vi "Leggi perdite di carico.vi"(4 "Lungh tubo asp":dbl, 5 "Dia ASP":string, 6 "Enum":T1(ring), 7 "Dia mand":string, 8 "PORTATA":dbl, 9 "DIAMETRO MAND ASP":i16, 10 "TAGLIA":string, 11 "SERIE":string) -> (0 "Perdite carico Mandata":dbl, 1 "Perdite carico Misura":dbl, 2 "Perdite carico MAND":dbl, 3 "Perdite carico ASP":dbl)   [LabVIEW 2019]
uses:
  Global percorso impostazioni.vi
panel:
  in  "Excel._Worksheet 15":refnum<k7>
  in  "Excel._Worksheet 14":refnum<k7>
  in  "Excel._Worksheet 13":refnum<k7>
  in  "Excel._Worksheet 12":refnum<k7>
  in  "Excel._Worksheet 10":refnum<k7>
  in  "Excel._Worksheet 4":refnum<k7>
  in  "WindowState 3":i32(ring)=-4137 items=["xlMaximized"=-4137, "xlMinimized"=-4140, "xlNormal"=-4143]
  out "error out 2":errorcluster
  in  "Excel._Worksheet 9":refnum<k7>
  in  "Excel._Worksheet 8":refnum<k7>
  out "error out":errorcluster
  in  "Excel._Worksheet 7":refnum<k7>
  in  "Excel._Worksheet 6":refnum<k7>
  in  "Excel._Worksheet 5":refnum<k7>
  in  "Excel._Worksheet 3":refnum<k7>
  in  "Excel._Worksheet 2":refnum<k7>
  in  "WindowState 2":i32(ring)=-4137 items=["xlMaximized"=-4137, "xlMinimized"=-4140, "xlNormal"=-4143]
  # "pompe di superficie"
  # "pompe di verticali\\sommerse"
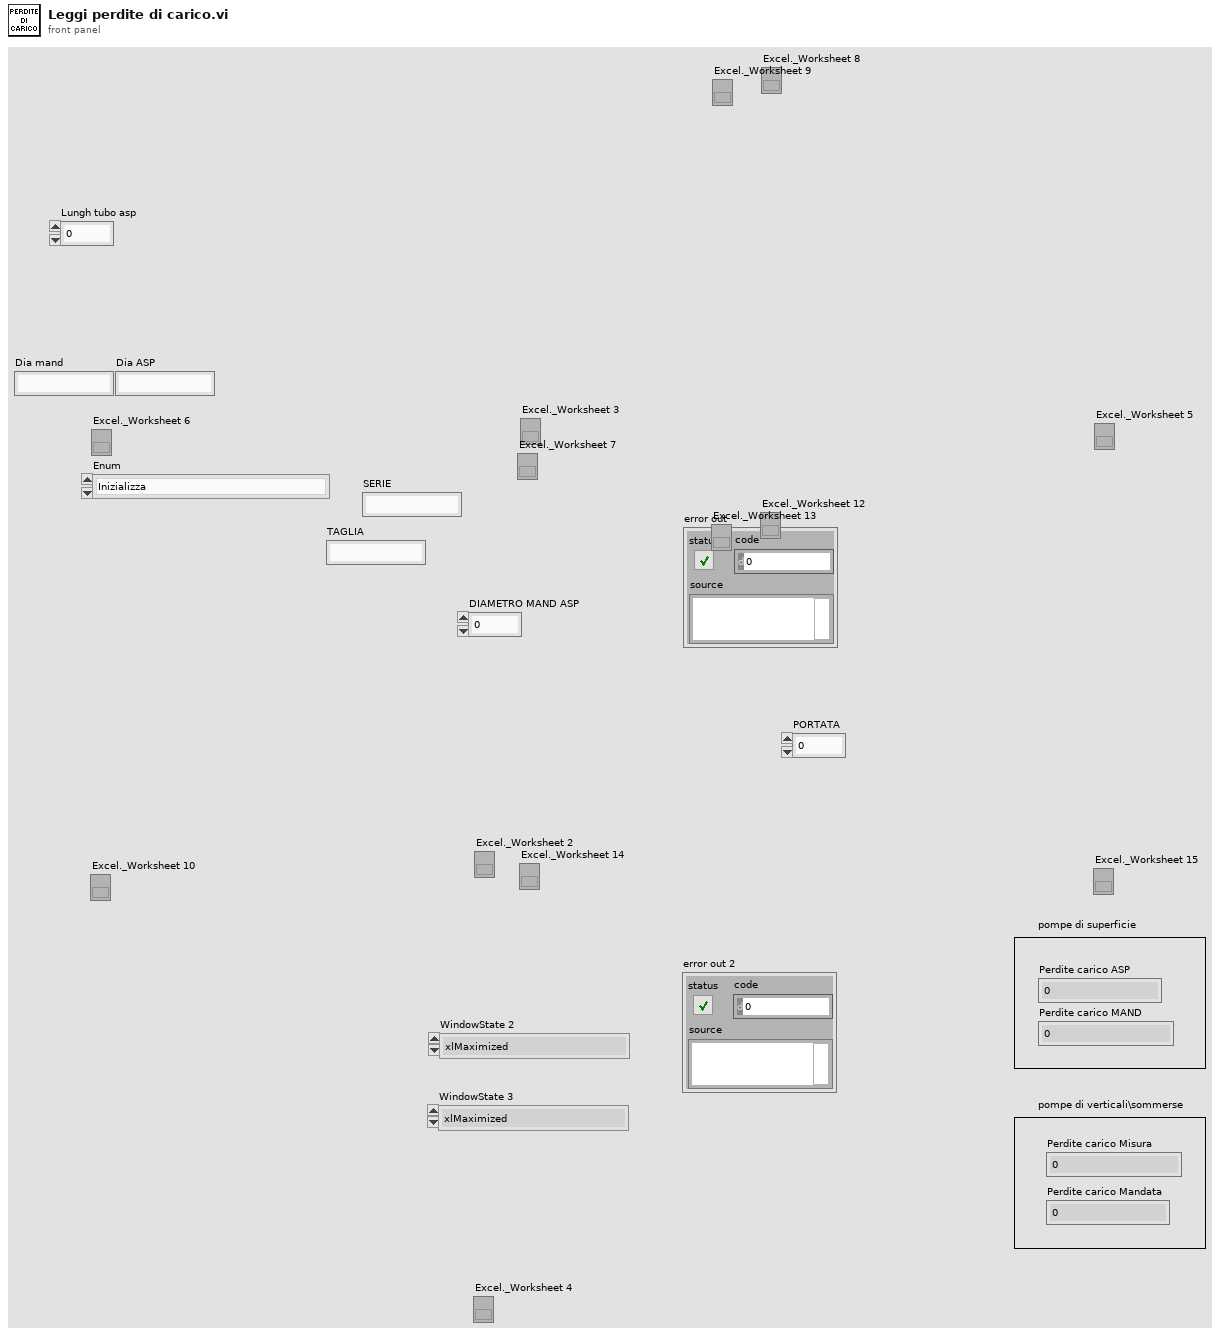
[diagram p1: front panel]
types:
  T1 = enum16{"Inizializza", "Imposta selezioni pompa", "Leggi perdite", "Close"}
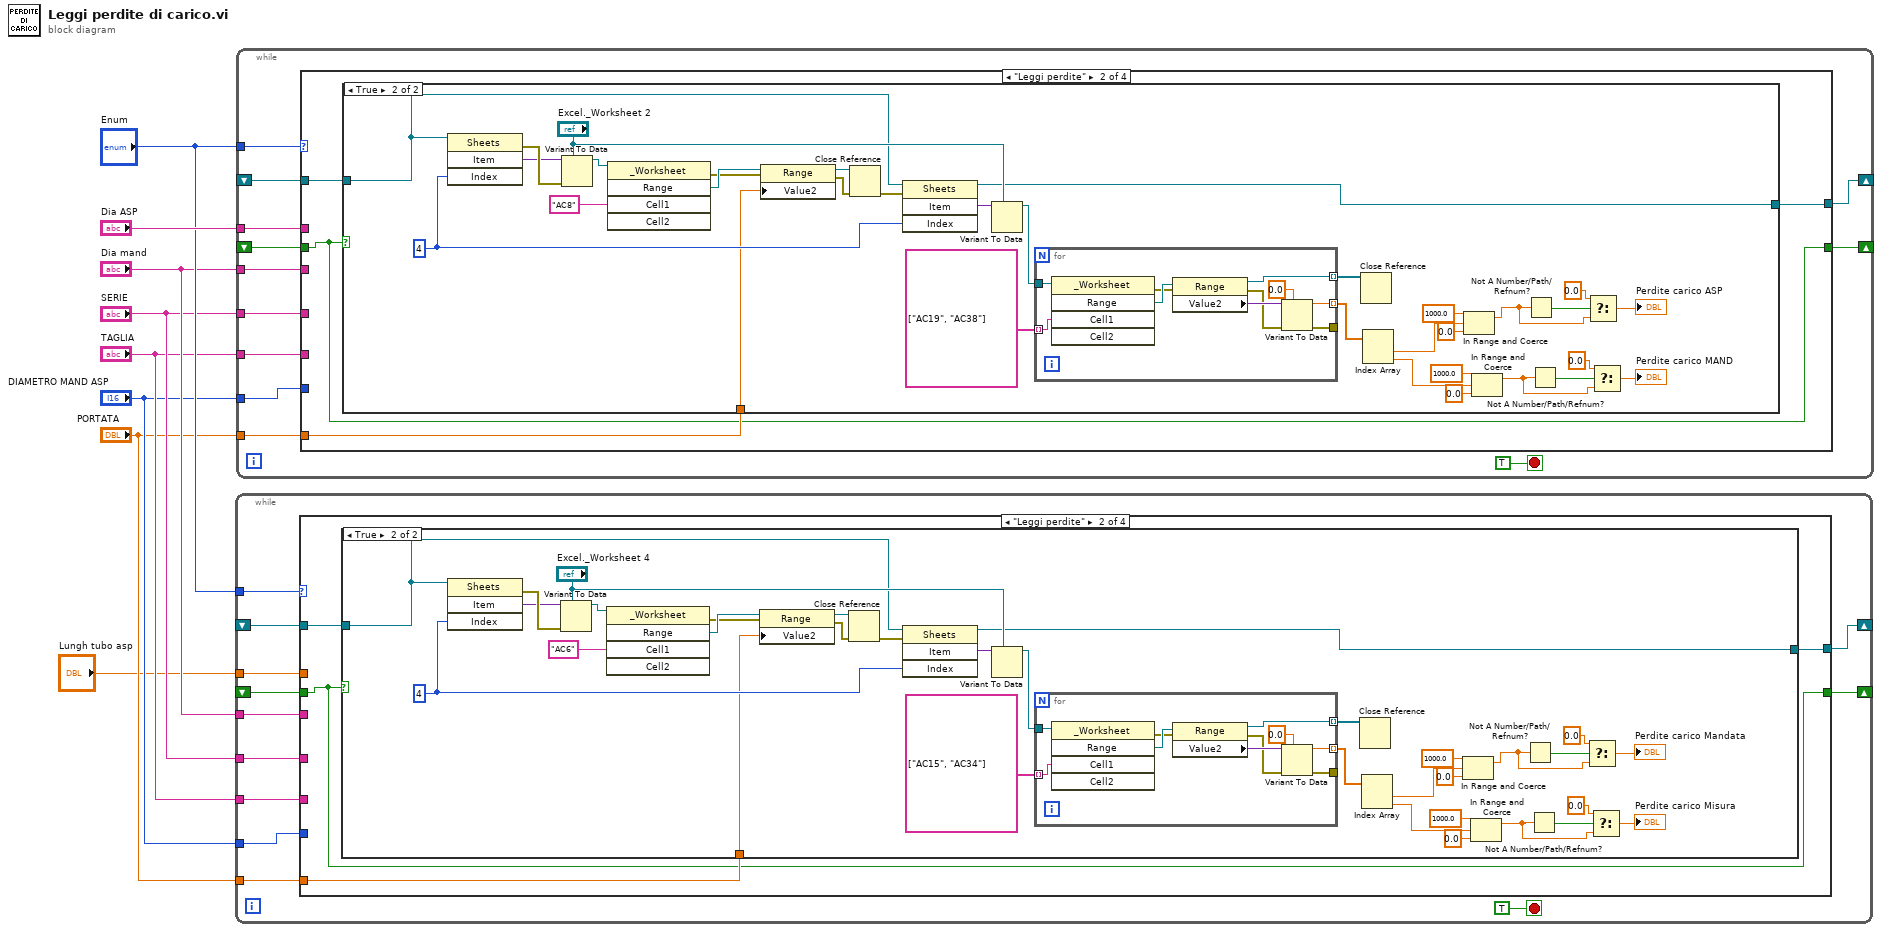
[diagram p0: block diagram]
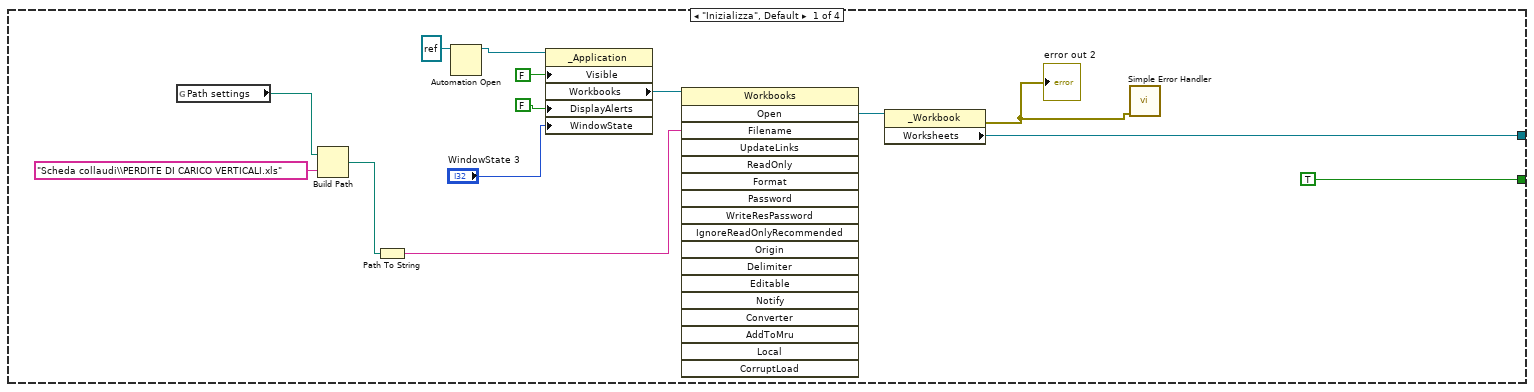
[diagram p2: hidden frame]
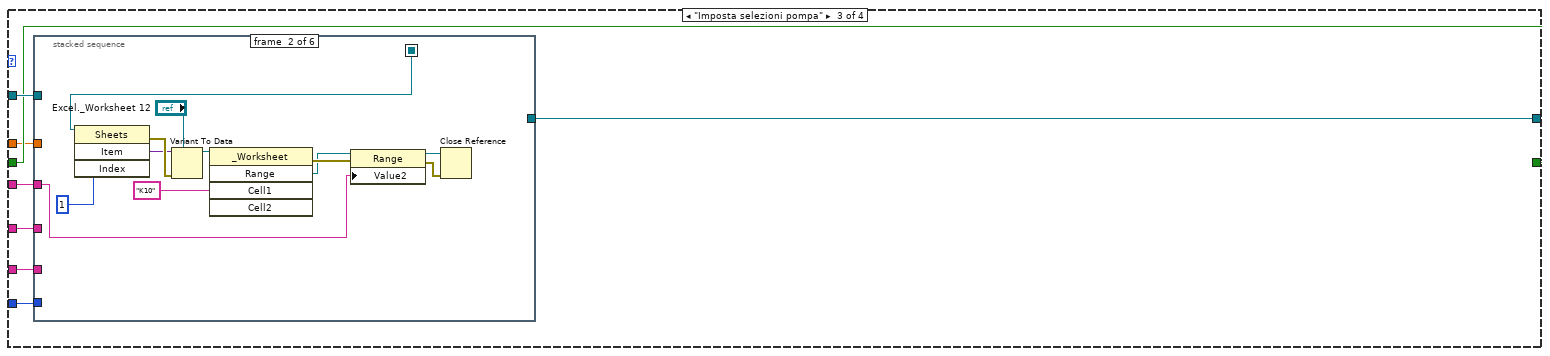
[diagram p4: hidden frame]
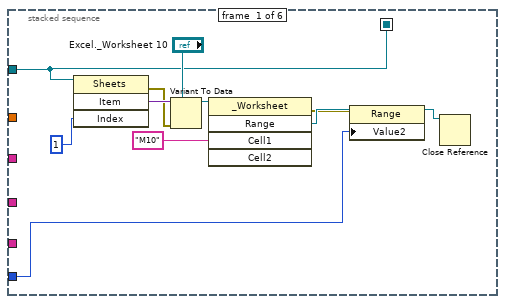
[diagram p5: hidden frame]
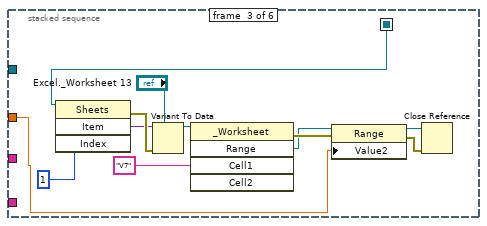
[diagram p6: hidden frame]
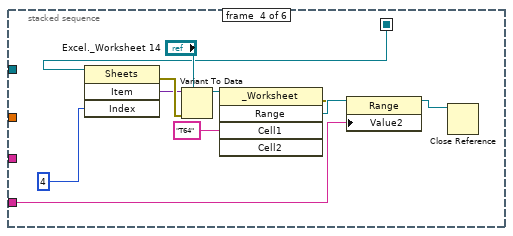
[diagram p7: hidden frame]
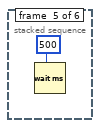
[diagram p8: hidden frame]
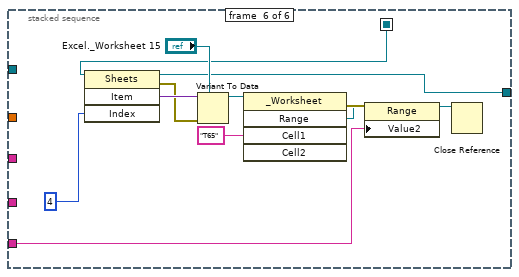
[diagram p9: hidden frame]
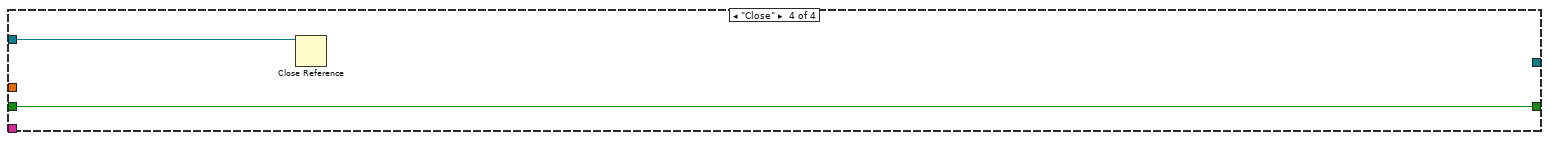
[diagram p10: hidden frame]
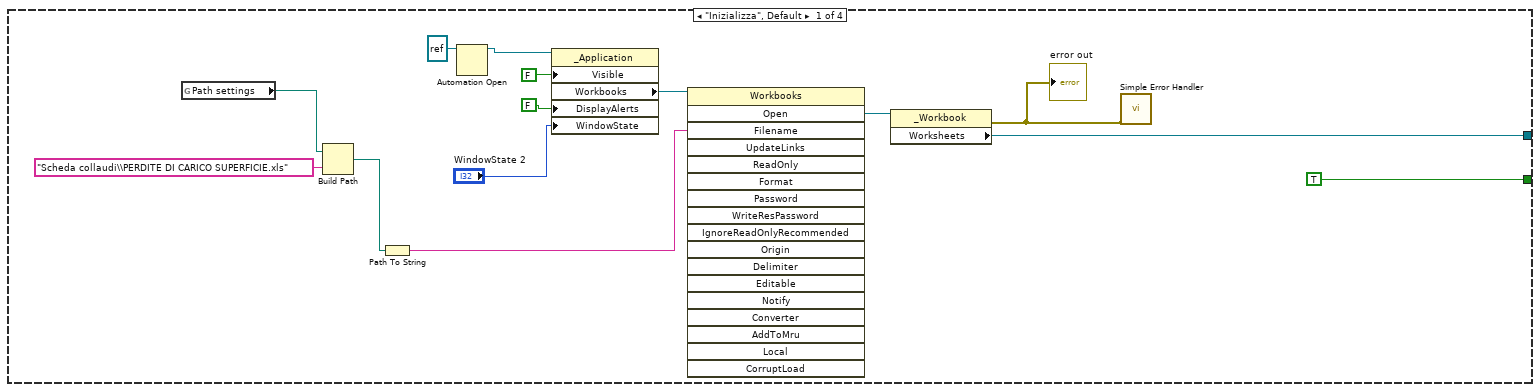
[diagram p11: hidden frame]
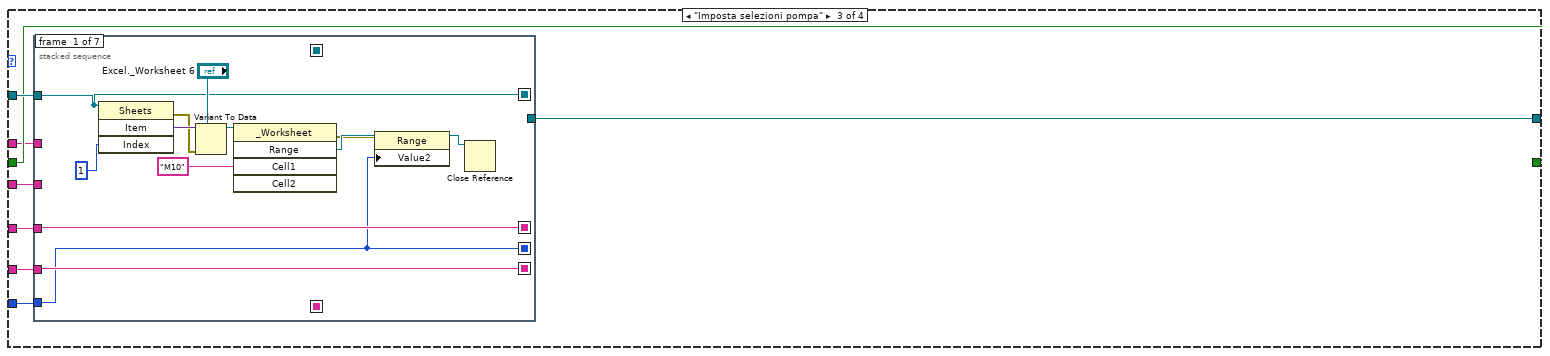
[diagram p13: hidden frame]
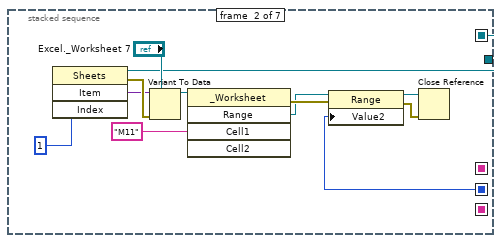
[diagram p14: hidden frame]
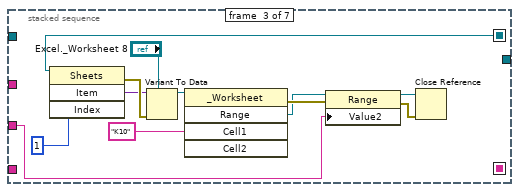
[diagram p15: hidden frame]
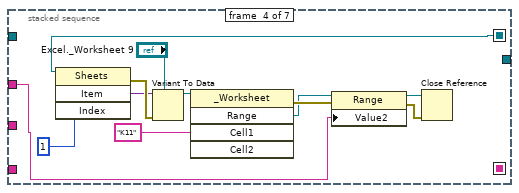
[diagram p16: hidden frame]
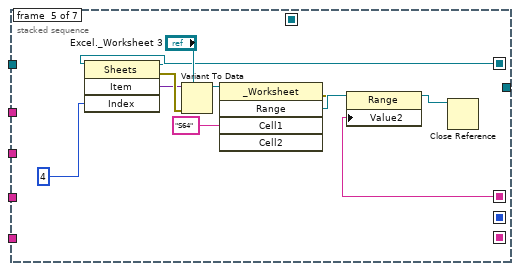
[diagram p17: hidden frame]
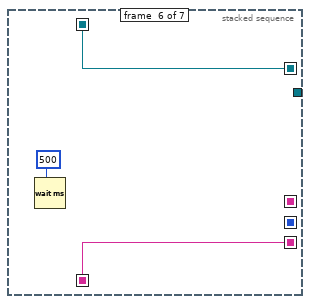
[diagram p18: hidden frame]
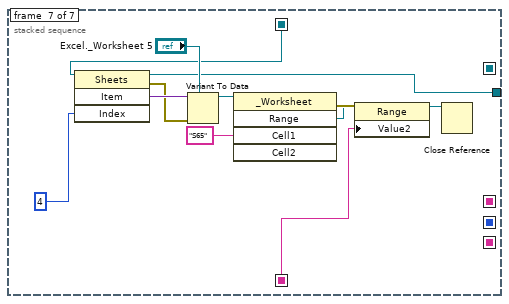
[diagram p19: hidden frame]
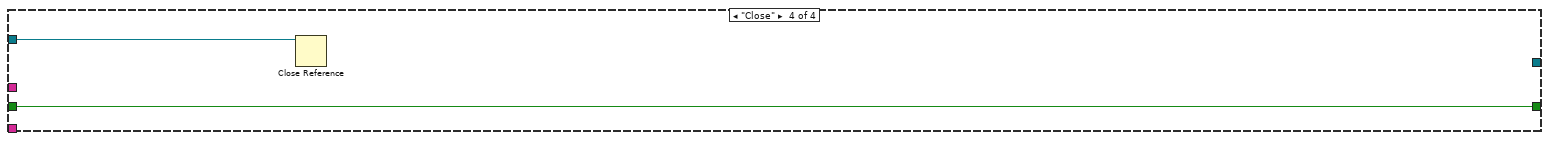
[diagram p20: hidden frame]
diagram:
  n1 = while {
    shift-right: [w19] -> _
    shift-left: _ -> [w18]
    tunnel: "SERIE" -> [w17]
    tunnel: "TAGLIA" -> [w16]
    tunnel: "DIAMETRO MAND ASP" -> [w15]
    tunnel: "Enum" -> [w14]
    tunnel: "PORTATA" -> [w13]
    shift-right: [w12] -> _
    shift-left: _ -> [w11]
    tunnel: "Dia mand" -> [w10]
    tunnel: "Lungh tubo asp" -> [w9]
    stop <- TRUE stop-if-true
    n2 = case shown="\"Leggi perdite\"" w14 {
      tunnel: [w23 w37 w86 _] -> w19
      tunnel: w18 -> [_ w38 w90 w151]
      tunnel: w17 -> [_ _ w89 _]
      tunnel: w16 -> [_ _ w88 _]
      tunnel: w15 -> [_ _ w87 _]
      tunnel: w13 -> [_ w36 _ _]
      tunnel: [TRUE w35 w85 w150] -> w12
      tunnel: w11 -> [_ w35 w85 w150]
      tunnel: w10 -> [_ _ w84 _]
      tunnel: w9 -> [_ _ w83 _]
      frame "Inizializza", Default {
        n3 = global read "Global percorso impostazioni.vi" "Path settings"() -> (w27:path)
        n4 = Build Path(base path=w27, name or relative path="Scheda collaudi\\PERDITE DI CARICO VERTICALI.xls") -> (appended path=w25:path)
        n5 = Path To String(path=w25) -> (string=w33:string)
        n6 = Automation Open(Automation Refnum=refnum<k7> refnum ("Excel._Application")) -> (Automation Refnum=w34:refnum<k7>)  [unwired: 3 in, 1 out]
        n7 = property class="_Application"(reference=w34, "Visible"=FALSE, "DisplayAlerts"=FALSE, "WindowState"="WindowState 3") -> ("Workbooks"=w22:refnum<k7>)  [unwired: 1 in, 2 out]
        n8 = invoke class="Workbooks" method="Open"(reference=w22, "Filename"=w33) -> ("Open"=w24:refnum<k7>)  [unwired: 16 in, 17 out]
        n9 = property class="_Workbook"(reference=w24) -> (error out=w21:errorcluster, "Worksheets"=w23:refnum<k7>)  [unwired: 1 in, 1 out]
        "error out 2" <- w21
        n10 = call <vilib>:"Simple Error Handler.vi"("error in (no error)"=w21) -> ()  [unwired: 4 in, 5 out]
      }
      frame "Leggi perdite" {
        n11 = case shown="True" w35 {
          tunnel: w38 -> [w39 w58]
          tunnel: [w39 w57] -> w37
          tunnel: w36 -> [_ w40]
          frame False {
          }
          frame True {
            w64 = 4 ("Sheet Index")
            n12 = invoke class="Sheets" method="Item"(reference=w58, "Index"=w64) -> (error out=w60:errorcluster, "Item"=w59:variant)  [unwired: 2 in, 2 out]
            n13 = Variant To Data(error in=w60, type="Excel._Worksheet 4", Variant=w59) -> (data=w62:refnum<k7>)  [unwired: 1 out]
            n14 = invoke class="_Worksheet" method="Range"(reference=w62, "Cell1"="AC6") -> (error out=w65:errorcluster, "Range"=w66:refnum<k7>)  [unwired: 3 in, 3 out]
            n15 = property class="Range"(reference=w66, error in=w65, "Value2"=w40) -> (reference out=w70:refnum<k7>, error out=w71:errorcluster)
            n16 = Close Reference(reference=w70, error in (no error)=w71) -> (error out=w72:errorcluster)
            n17 = invoke class="Sheets" method="Item"(reference=w58, error in=w72, "Index"=w64) -> (reference out=w57:refnum<k7>, "Item"=w63:variant)  [unwired: 1 in, 2 out]
            n18 = Variant To Data(type="Excel._Worksheet 4", Variant=w63) -> (data=w69:refnum<k7>)  [unwired: 1 in, 1 out]
            n19 = for {
              tunnel: w69 -> [w82]
              tunnel: [w77] -> w55 mode=indexing
              tunnel: string[] ["AC15", "AC34"] -> [w76] mode=indexing
              tunnel: [w74] -> _
              tunnel: [w73] -> w56 mode=indexing
              n20 = invoke class="_Worksheet" method="Range"(reference=w82, "Cell1"=w76) -> (error out=w80:errorcluster, "Range"=w81:refnum<k7>)  [unwired: 3 in, 3 out]
              n21 = property class="Range"(reference=w81, error in=w80) -> (reference out=w73:refnum<k7>, error out=w78:errorcluster, "Value2"=w79:variant)
              n22 = Variant To Data(error in=w78, type=0.0, Variant=w79) -> (data=w77:dbl, error out=w74:errorcluster)
            }
            n23 = Close Reference(reference=w56) -> ()  [unwired: 1 in, 1 out]
            n24 = Index Array(array=w55) -> (element #1=w54:dbl, element #2=w49:dbl)  [unwired: 2 in]
            n25 = In Range and Coerce(upper limit=1000.0, x=w54, lower limit=0.0) -> (coerced(x)=w46:dbl)  [unwired: 1 out]
            n26 = In Range and Coerce(upper limit=1000.0, x=w49, lower limit=0.0) -> (coerced(x)=w42:dbl)  [unwired: 1 out]
            n27 = Not A Number/Path/Refnum?(number/path/refnum=w46) -> (NaN/Path/Refnum?=w48:bool)
            n28 = Not A Number/Path/Refnum?(number/path/refnum=w42) -> (NaN/Path/Refnum?=w43:bool)
            n29 = Select(t=0.0, s=w48, f=w46) -> (s? t:f=→"Perdite carico Mandata":dbl)
            n30 = Select(t=0.0, s=w43, f=w42) -> (s? t:f=→"Perdite carico Misura":dbl)
          }
        }
      }
      frame "Imposta selezioni pompa" {
        n31 = stacked-sequence {
          seq-local: [w91 _ _ _ _ _] -> [_ w102 w114 w126 _ w141]
          tunnel: w90 -> [w91 _ _ _ _ _]
          tunnel: w89 -> [_ _ _ w127 _ _]
          tunnel: w88 -> [_ _ _ _ _ w138]
          tunnel: w87 -> [w93 _ _ _ _ _]
          tunnel: [_ _ _ _ _ w140] -> w86
          tunnel: w84 -> [_ w103 _ _ _ _]
          tunnel: w83 -> [_ _ w115 _ _ _]
          frame #0 {
            n32 = invoke class="Sheets" method="Item"(reference=w91, "Index"=1 ("Sheet Index")) -> (error out=w100:errorcluster, "Item"=w101:variant)  [unwired: 2 in, 2 out]
            n33 = Variant To Data(error in=w100, type="Excel._Worksheet 10", Variant=w101) -> (data=w94:refnum<k7>)  [unwired: 1 out]
            n34 = invoke class="_Worksheet" method="Range"(reference=w94, "Cell1"="M10") -> (error out=w95:errorcluster, "Range"=w99:refnum<k7>)  [unwired: 3 in, 3 out]
            n35 = property class="Range"(reference=w99, error in=w95, "Value2"=w93) -> (reference out=w92:refnum<k7>)  [unwired: 1 out]
            n36 = Close Reference(reference=w92) -> ()  [unwired: 1 in, 1 out]
          }
          frame #1 {
            n37 = invoke class="Sheets" method="Item"(reference=w102, "Index"=1 ("Sheet Index")) -> (error out=w107:errorcluster, "Item"=w106:variant)  [unwired: 2 in, 2 out]
            n38 = Variant To Data(error in=w107, type="Excel._Worksheet 12", Variant=w106) -> (data=w113:refnum<k7>)  [unwired: 1 out]
            n39 = invoke class="_Worksheet" method="Range"(reference=w113, "Cell1"="K10") -> (error out=w112:errorcluster, "Range"=w108:refnum<k7>)  [unwired: 3 in, 3 out]
            n40 = property class="Range"(reference=w108, error in=w112, "Value2"=w103) -> (reference out=w104:refnum<k7>, error out=w105:errorcluster)
            n41 = Close Reference(reference=w104, error in (no error)=w105) -> ()  [unwired: 1 out]
          }
          frame #2 {
            n42 = invoke class="Sheets" method="Item"(reference=w114, "Index"=1 ("Sheet Index")) -> (error out=w119:errorcluster, "Item"=w118:variant)  [unwired: 2 in, 2 out]
            n43 = Variant To Data(error in=w119, type="Excel._Worksheet 13", Variant=w118) -> (data=w125:refnum<k7>)  [unwired: 1 out]
            n44 = invoke class="_Worksheet" method="Range"(reference=w125, "Cell1"="V7") -> (error out=w124:errorcluster, "Range"=w120:refnum<k7>)  [unwired: 3 in, 3 out]
            n45 = property class="Range"(reference=w120, error in=w124, "Value2"=w115) -> (reference out=w116:refnum<k7>, error out=w117:errorcluster)
            n46 = Close Reference(reference=w116, error in (no error)=w117) -> ()  [unwired: 1 out]
          }
          frame #3 {
            n47 = invoke class="Sheets" method="Item"(reference=w126, "Index"=4 ("Sheet Index")) -> (error out=w131:errorcluster, "Item"=w130:variant)  [unwired: 2 in, 2 out]
            n48 = Variant To Data(error in=w131, type="Excel._Worksheet 14", Variant=w130) -> (data=w132:refnum<k7>)  [unwired: 1 out]
            n49 = invoke class="_Worksheet" method="Range"(reference=w132, "Cell1"="T64") -> (error out=w133:errorcluster, "Range"=w134:refnum<k7>)  [unwired: 3 in, 3 out]
            n50 = property class="Range"(reference=w134, error in=w133, "Value2"=w127) -> (reference out=w128:refnum<k7>)  [unwired: 1 out]
            n51 = Close Reference(reference=w128) -> ()  [unwired: 1 in, 1 out]
          }
          frame #4 {
            n52 = Wait (ms)(milliseconds to wait=u32 500) -> ()  [unwired: 1 out]
          }
          frame #5 {
            n53 = invoke class="Sheets" method="Item"(reference=w141, "Index"=4 ("Sheet Index")) -> (reference out=w140:refnum<k7>, error out=w147:errorcluster, "Item"=w148:variant)  [unwired: 2 in, 1 out]
            n54 = Variant To Data(error in=w147, type="Excel._Worksheet 15", Variant=w148) -> (data=w146:refnum<k7>)  [unwired: 1 out]
            n55 = invoke class="_Worksheet" method="Range"(reference=w146, "Cell1"="T65") -> (error out=w145:errorcluster, "Range"=w144:refnum<k7>)  [unwired: 3 in, 3 out]
            n56 = property class="Range"(reference=w144, error in=w145, "Value2"=w138) -> (reference out=w139:refnum<k7>)  [unwired: 1 out]
            n57 = Close Reference(reference=w139) -> ()  [unwired: 1 in, 1 out]
          }
        }
      }
      frame "Close" {
        n58 = Close Reference(reference=w151) -> ()  [unwired: 1 in, 1 out]
      }
    }
  }
  n59 = while {
    shift-right: [w162] -> _
    shift-left: _ -> [w161]
    tunnel: "SERIE" -> [w160]
    tunnel: "TAGLIA" -> [w159]
    tunnel: "DIAMETRO MAND ASP" -> [w158]
    tunnel: "Enum" -> [w157]
    tunnel: "PORTATA" -> [w156]
    shift-right: [w155] -> _
    shift-left: _ -> [w154]
    tunnel: "Dia mand" -> [w153]
    tunnel: "Dia ASP" -> [w152]
    stop <- TRUE stop-if-true
    n60 = case shown="\"Leggi perdite\"" w157 {
      tunnel: [w166 w180 w229 _] -> w162
      tunnel: w161 -> [_ w181 w233 w314]
      tunnel: w160 -> [_ _ w232 _]
      tunnel: w159 -> [_ _ w231 _]
      tunnel: w158 -> [_ _ w230 _]
      tunnel: w156 -> [_ w179 _ _]
      tunnel: [TRUE w178 w228 w313] -> w155
      tunnel: w154 -> [_ w178 w228 w313]
      tunnel: w153 -> [_ _ w227 _]
      tunnel: w152 -> [_ _ w226 _]
      frame "Inizializza", Default {
        n61 = global read "Global percorso impostazioni.vi" "Path settings"() -> (w170:path)
        n62 = Build Path(base path=w170, name or relative path="Scheda collaudi\\PERDITE DI CARICO SUPERFICIE.xls") -> (appended path=w168:path)
        n63 = Path To String(path=w168) -> (string=w176:string)
        n64 = Automation Open(Automation Refnum=refnum<k7> refnum ("Excel._Application")) -> (Automation Refnum=w177:refnum<k7>)  [unwired: 3 in, 1 out]
        n65 = property class="_Application"(reference=w177, "Visible"=FALSE, "DisplayAlerts"=FALSE, "WindowState"="WindowState 2") -> ("Workbooks"=w165:refnum<k7>)  [unwired: 1 in, 2 out]
        n66 = invoke class="Workbooks" method="Open"(reference=w165, "Filename"=w176) -> ("Open"=w167:refnum<k7>)  [unwired: 16 in, 17 out]
        n67 = property class="_Workbook"(reference=w167) -> (error out=w164:errorcluster, "Worksheets"=w166:refnum<k7>)  [unwired: 1 in, 1 out]
        "error out" <- w164
        n68 = call <vilib>:"Simple Error Handler.vi"("error in (no error)"=w164) -> ()  [unwired: 4 in, 5 out]
      }
      frame "Leggi perdite" {
        n69 = case shown="True" w178 {
          tunnel: w181 -> [w182 w201]
          tunnel: [w182 w200] -> w180
          tunnel: w179 -> [_ w183]
          frame False {
          }
          frame True {
            w207 = 4 ("Sheet Index")
            n70 = invoke class="Sheets" method="Item"(reference=w201, "Index"=w207) -> (error out=w203:errorcluster, "Item"=w202:variant)  [unwired: 2 in, 2 out]
            n71 = Variant To Data(error in=w203, type="Excel._Worksheet 2", Variant=w202) -> (data=w205:refnum<k7>)  [unwired: 1 out]
            n72 = invoke class="_Worksheet" method="Range"(reference=w205, "Cell1"="AC8") -> (error out=w208:errorcluster, "Range"=w209:refnum<k7>)  [unwired: 3 in, 3 out]
            n73 = property class="Range"(reference=w209, error in=w208, "Value2"=w183) -> (reference out=w213:refnum<k7>, error out=w214:errorcluster)
            n74 = Close Reference(reference=w213, error in (no error)=w214) -> (error out=w215:errorcluster)
            n75 = invoke class="Sheets" method="Item"(reference=w201, error in=w215, "Index"=w207) -> (reference out=w200:refnum<k7>, "Item"=w206:variant)  [unwired: 1 in, 2 out]
            n76 = Variant To Data(type="Excel._Worksheet 2", Variant=w206) -> (data=w212:refnum<k7>)  [unwired: 1 in, 1 out]
            n77 = for {
              tunnel: w212 -> [w225]
              tunnel: [w220] -> w198 mode=indexing
              tunnel: string[] ["AC19", "AC38"] -> [w219] mode=indexing
              tunnel: [w217] -> _
              tunnel: [w216] -> w199 mode=indexing
              n78 = invoke class="_Worksheet" method="Range"(reference=w225, "Cell1"=w219) -> (error out=w223:errorcluster, "Range"=w224:refnum<k7>)  [unwired: 3 in, 3 out]
              n79 = property class="Range"(reference=w224, error in=w223) -> (reference out=w216:refnum<k7>, error out=w221:errorcluster, "Value2"=w222:variant)
              n80 = Variant To Data(error in=w221, type=0.0, Variant=w222) -> (data=w220:dbl, error out=w217:errorcluster)
            }
            n81 = Close Reference(reference=w199) -> ()  [unwired: 1 in, 1 out]
            n82 = Index Array(array=w198) -> (element #1=w197:dbl, element #2=w192:dbl)  [unwired: 2 in]
            n83 = In Range and Coerce(upper limit=1000.0, x=w197, lower limit=0.0) -> (coerced(x)=w189:dbl)  [unwired: 1 out]
            n84 = In Range and Coerce(upper limit=1000.0, x=w192, lower limit=0.0) -> (coerced(x)=w185:dbl)  [unwired: 1 out]
            n85 = Not A Number/Path/Refnum?(number/path/refnum=w189) -> (NaN/Path/Refnum?=w191:bool)
            n86 = Not A Number/Path/Refnum?(number/path/refnum=w185) -> (NaN/Path/Refnum?=w186:bool)
            n87 = Select(t=0.0, s=w191, f=w189) -> (s? t:f=→"Perdite carico ASP":dbl)
            n88 = Select(t=0.0, s=w186, f=w185) -> (s? t:f=→"Perdite carico MAND":dbl)
          }
        }
      }
      frame "Imposta selezioni pompa" {
        n89 = stacked-sequence {
          seq-local: [w239 _ _ _ _ _ _] -> [_ w250 w262 w274 _ _ _]
          seq-local: [w246 _ _ _ _ _ _] -> [_ w260 _ _ _ _ _]
          seq-local: [w245 _ _ _ _ _ _] -> [_ w259 _ _ _ _ _]
          seq-local: [w235 _ _ _ _ _ _] -> [_ w249 _ _ _ _ _]
          seq-local: [_ w250 _ _ _ _ _] -> [_ _ _ _ w290 _ _]
          seq-local: [_ w260 _ _ _ _ _] -> [_ _ _ _ w288 _ _]
          seq-local: [_ w259 _ _ _ _ _] -> [_ _ _ _ w287 _ _]
          seq-local: [_ _ _ _ w285 _ _] -> [_ _ _ _ _ w299 _]
          seq-local: [_ _ _ _ w287 _ _] -> [_ _ _ _ _ w298 _]
          seq-local: [_ _ _ _ _ w299 _] -> [_ _ _ _ _ _ w304]
          seq-local: [_ _ _ _ _ w298 _] -> [_ _ _ _ _ _ w303]
          tunnel: w233 -> [w239 _ _ _ _ _ _]
          tunnel: w232 -> [w246 _ _ _ _ _ _]
          tunnel: w231 -> [w245 _ _ _ _ _ _]
          tunnel: w230 -> [w235 _ _ _ _ _ _]
          tunnel: [_ _ _ _ _ _ w302] -> w229
          tunnel: w227 -> [_ _ w261 _ _ _ _]
          tunnel: w226 -> [_ _ _ w273 _ _ _]
          frame #0 {
            n90 = invoke class="Sheets" method="Item"(reference=w239, "Index"=1 ("Sheet Index")) -> (error out=w243:errorcluster, "Item"=w244:variant)  [unwired: 2 in, 2 out]
            n91 = Variant To Data(error in=w243, type="Excel._Worksheet 6", Variant=w244) -> (data=w236:refnum<k7>)  [unwired: 1 out]
            n92 = invoke class="_Worksheet" method="Range"(reference=w236, "Cell1"="M10") -> (error out=w237:errorcluster, "Range"=w242:refnum<k7>)  [unwired: 3 in, 3 out]
            n93 = property class="Range"(reference=w242, error in=w237, "Value2"=w235) -> (reference out=w234:refnum<k7>)  [unwired: 1 out]
            n94 = Close Reference(reference=w234) -> ()  [unwired: 1 in, 1 out]
          }
          frame #1 {
            n95 = invoke class="Sheets" method="Item"(reference=w250, "Index"=1 ("Sheet Index")) -> (error out=w252:errorcluster, "Item"=w251:variant)  [unwired: 2 in, 2 out]
            n96 = Variant To Data(error in=w252, type="Excel._Worksheet 7", Variant=w251) -> (data=w258:refnum<k7>)  [unwired: 1 out]
            n97 = invoke class="_Worksheet" method="Range"(reference=w258, "Cell1"="M11") -> (error out=w257:errorcluster, "Range"=w253:refnum<k7>)  [unwired: 3 in, 3 out]
            n98 = property class="Range"(reference=w253, error in=w257, "Value2"=w249) -> (reference out=w247:refnum<k7>, error out=w248:errorcluster)
            n99 = Close Reference(reference=w247, error in (no error)=w248) -> ()  [unwired: 1 out]
          }
          frame #2 {
            n100 = invoke class="Sheets" method="Item"(reference=w262, "Index"=1 ("Sheet Index")) -> (error out=w266:errorcluster, "Item"=w265:variant)  [unwired: 2 in, 2 out]
            n101 = Variant To Data(error in=w266, type="Excel._Worksheet 8", Variant=w265) -> (data=w272:refnum<k7>)  [unwired: 1 out]
            n102 = invoke class="_Worksheet" method="Range"(reference=w272, "Cell1"="K10") -> (error out=w271:errorcluster, "Range"=w267:refnum<k7>)  [unwired: 3 in, 3 out]
            n103 = property class="Range"(reference=w267, error in=w271, "Value2"=w261) -> (reference out=w263:refnum<k7>, error out=w264:errorcluster)
            n104 = Close Reference(reference=w263, error in (no error)=w264) -> ()  [unwired: 1 out]
          }
          frame #3 {
            n105 = invoke class="Sheets" method="Item"(reference=w274, "Index"=1 ("Sheet Index")) -> (error out=w278:errorcluster, "Item"=w277:variant)  [unwired: 2 in, 2 out]
            n106 = Variant To Data(error in=w278, type="Excel._Worksheet 9", Variant=w277) -> (data=w284:refnum<k7>)  [unwired: 1 out]
            n107 = invoke class="_Worksheet" method="Range"(reference=w284, "Cell1"="K11") -> (error out=w283:errorcluster, "Range"=w279:refnum<k7>)  [unwired: 3 in, 3 out]
            n108 = property class="Range"(reference=w279, error in=w283, "Value2"=w273) -> (reference out=w275:refnum<k7>, error out=w276:errorcluster)
            n109 = Close Reference(reference=w275, error in (no error)=w276) -> ()  [unwired: 1 out]
          }
          frame #4 {
            n110 = invoke class="Sheets" method="Item"(reference=w290, "Index"=4 ("Sheet Index")) -> (reference out=w285:refnum<k7>, error out=w292:errorcluster, "Item"=w291:variant)  [unwired: 2 in, 1 out]
            n111 = Variant To Data(error in=w292, type="Excel._Worksheet 3", Variant=w291) -> (data=w293:refnum<k7>)  [unwired: 1 out]
            n112 = invoke class="_Worksheet" method="Range"(reference=w293, "Cell1"="S64") -> (error out=w294:errorcluster, "Range"=w295:refnum<k7>)  [unwired: 3 in, 3 out]
            n113 = property class="Range"(reference=w295, error in=w294, "Value2"=w288) -> (reference out=w286:refnum<k7>)  [unwired: 1 out]
            n114 = Close Reference(reference=w286) -> ()  [unwired: 1 in, 1 out]
          }
          frame #5 {
            n115 = Wait (ms)(milliseconds to wait=u32 500) -> ()  [unwired: 1 out]
          }
          frame #6 {
            n116 = invoke class="Sheets" method="Item"(reference=w304, "Index"=4 ("Sheet Index")) -> (reference out=w302:refnum<k7>, error out=w310:errorcluster, "Item"=w311:variant)  [unwired: 2 in, 1 out]
            n117 = Variant To Data(error in=w310, type="Excel._Worksheet 5", Variant=w311) -> (data=w309:refnum<k7>)  [unwired: 1 out]
            n118 = invoke class="_Worksheet" method="Range"(reference=w309, "Cell1"="S65") -> (error out=w308:errorcluster, "Range"=w307:refnum<k7>)  [unwired: 3 in, 3 out]
            n119 = property class="Range"(reference=w307, error in=w308, "Value2"=w303) -> (reference out=w301:refnum<k7>)  [unwired: 1 out]
            n120 = Close Reference(reference=w301) -> ()  [unwired: 1 in, 1 out]
          }
        }
      }
      frame "Close" {
        n121 = Close Reference(reference=w314) -> ()  [unwired: 1 in, 1 out]
      }
    }
  }
